vi "NATS Client Integration Test.vi"() -> (0 "error out":errorcluster)   [LabVIEW 2024]
uses:
  <vilib>/addons/_JKI Toolkits/Caraya/classes/Assert/Assert False.vi
  <vilib>/addons/_JKI Toolkits/Caraya/classes/Assert/Assert Equal Value and Type_Variant.vi
  NATS Subscription/NATS Subscription.lvclass
  <vilib>/addons/_JKI Toolkits/Caraya/classes/Test/Test.lvclass
  NATS Client/NATS Client.lvclass
  <vilib>/addons/_JKI Toolkits/Caraya/classes/Assert/Assert.lvclass
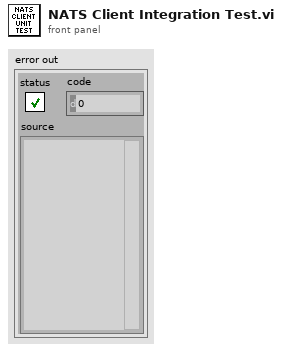
[diagram p1: front panel]
types:
  T1 = typedef "NATS Core.lvlib/nats message.ctl" = cluster{"subject":string, "payload":string, "sub id":string, "reply-to":string, "headers":string, "type":T2, "received":timestamp}
  T2 = typedef "NATS Core.lvlib/msg type.ctl" = enum16{"Undefined", "MSG", "HMSG", "+OK", "PING", "PONG", "-ERR", "INFO"}
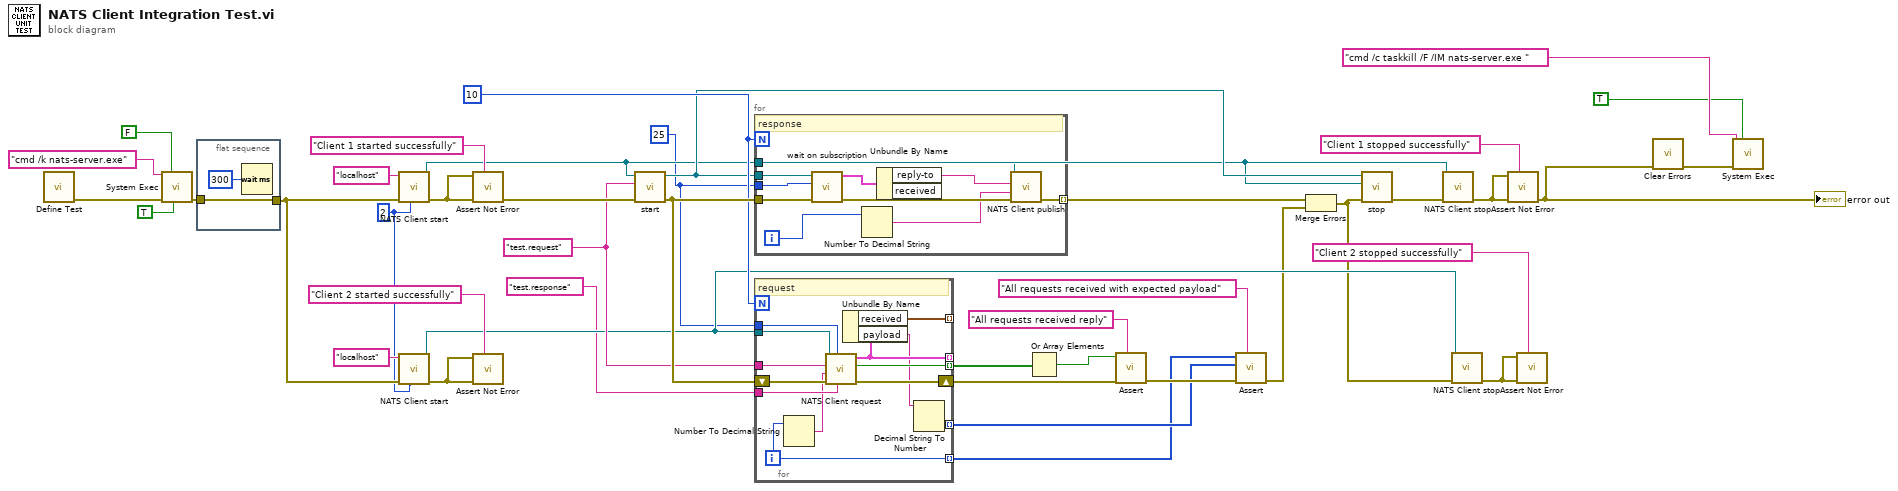
[diagram p0: block diagram]
diagram:
  w2 = 2 ("timeout ms (5)")
  w1 = 25 ("timeout in ms (-1)")
  w21 = 10
  w22 = "test.request"
  n1 = call <vilib>:"Define Test.vi"() -> ("error out"=w40:errorcluster)  [unwired: 10 in, 1 out]
  n2 = call <vilib>:"System Exec.vi"("run minimized? (F)"=TRUE, "wait until completion? (T)"=FALSE, "error in (no error)"=w40, "command line"="cmd /k nats-server.exe") -> ("error out"=w17:errorcluster)  [unwired: 4 in, 3 out]
  n3 = flat-sequence {
    tunnel: [w43] -> w16
    tunnel: w17 -> [w43]
    frame #0 {
      n4 = Wait (ms)(milliseconds to wait=u32 300) -> ()  [unwired: 1 out]
    }
  }
  n5 = call "NATS Client start.vi"("timeout ms (5)"=w2, "error in"=w16, "address"="localhost") -> ("error out"=w42:errorcluster, "NATS Client out"=w14:refnum<class "NATS Client.lvclass">)  [unwired: 7 in]
  n6 = call "NATS Client start.vi"("timeout ms (5)"=w2, "error in"=w16, "address"="localhost") -> ("error out"=w37:errorcluster, "NATS Client out"=w18:refnum<class "NATS Client.lvclass">)  [unwired: 7 in]
  n7 = call <vilib>:"Assert Not Error.vi"("Label"="Client 1 started successfully", "error in (no error)"=w42, "Not Error?"=w42) -> ("error out"=w36:errorcluster)  [unwired: 7 in, 1 out]
  n8 = call <vilib>:"Assert Not Error.vi"("Label"="Client 2 started successfully", "error in (no error)"=w37, "Not Error?"=w37) -> ()  [unwired: 7 in, 2 out]
  n9 = call "start.vi"("error in"=w36, "subject"=w22, "NATS Client"=w14) -> ("error out"=w33:errorcluster, "NATS Subscription"=w20:refnum<class "NATS Subscription.lvclass">)  [unwired: 7 in]
  n10 = for {
    N: w21 -> [_]
    tunnel: w20 -> [w53]
    tunnel: w14 -> [w51]
    tunnel: w1 -> [w45]
    tunnel: w33 -> [w54]
    tunnel: [w46] -> w11 mode=indexing
    i -> [w48]
    # "response"
    n11 = call-dynamic "wait on subscription.vi"("error in"=w54, "timeout in ms (-1)"=w45, "NATS Subscriber in"=w53) -> ("error out"=w52:errorcluster, "nats message"=w50:T1)  [unwired: 6 in, 1 out]
    n12 = Number To Decimal String(number=w48) -> (decimal integer string=w47:string)  [unwired: 1 in]
    n13 = Unbundle By Name(w50) -> ("reply-to"=w49:string)  [unwired: 1 out]
    n14 = call "NATS Client publish.vi"("error in"=w52, "payload"=w47, "subject"=w49, "NATS Client.lvlib:NATS Client.lvclass"=w51) -> ("error out"=w46:errorcluster)  [unwired: 7 in]
  }
  n15 = for {
    N: w21 -> [_]
    tunnel: w18 -> [w65]
    tunnel: w22 -> [w64]
    shift-right: [w66] -> w9
    shift-left: w33 -> [w67]
    tunnel: "test.response" -> [w63]
    tunnel: [w62] -> w13 mode=indexing
    tunnel: [w61] -> _ mode=indexing
    tunnel: [w58] -> w7 mode=indexing
    tunnel: [w57] -> w6 mode=indexing
    tunnel: [w56] -> _ mode=indexing
    tunnel: w1 -> [w55]
    i -> [w57]
    # "request"
    n16 = Number To Decimal String(number=w57) -> (decimal integer string=w60:string)  [unwired: 1 in]
    n17 = call "NATS Client request.vi"("reply subject"=w63, "timeout in ms (-1)"=w55, "error in"=w67, "payload"=w60, "subject"=w64, "NATS Client in"=w65) -> ("error out"=w66:errorcluster, "time out"=w62:bool, "nats message"=w61:T1)  [unwired: 3 in]
    n18 = Unbundle By Name(w61) -> ("received"=w56:timestamp, "payload"=w59:string)
    n19 = Decimal String To Number(string=w59) -> (number=w58:i32)  [unwired: 2 in, 1 out]
  }
  n20 = Or Array Elements(Boolean array=w13) -> (logical OR=w12:bool)
  n21 = call-poly <vilib>:"Assert.vi"("Label"="All requests received reply", "error in (no error)"=w9, "False?"=w12) -> ("error out"=w10:errorcluster)  [unwired: 7 in, 1 out]
  n22 = call-poly <vilib>:"Assert.vi"("Label"="All requests received with expected payload", "error in (no error)"=w10, "Y"=w7, "X"=w6) -> ("error out"=w4:errorcluster)  [unwired: 6 in, 1 out]
  n23 = Merge Errors(w11, w4) -> (w3:errorcluster)
  n24 = call "stop.vi"("error in"=w3, "NATS Client"=w14, "NATS Subscription"=w20) -> ("error out"=w35:errorcluster)  [unwired: 8 in]
  n25 = call "NATS Client stop.vi"("error in"=w35, "NATS Client"=w14) -> ("error out"=w41:errorcluster)  [unwired: 9 in]
  n26 = call "NATS Client stop.vi"("error in"=w3, "NATS Client"=w18) -> ("error out"=w34:errorcluster)  [unwired: 9 in]
  n27 = call <vilib>:"Assert Not Error.vi"("Label"="Client 1 stopped successfully", "error in (no error)"=w41, "Not Error?"=w41) -> ("error out"=w39:errorcluster)  [unwired: 7 in, 1 out]
  "error out" <- w39
  n28 = call <vilib>:"Assert Not Error.vi"("Label"="Client 2 stopped successfully", "error in (no error)"=w34, "Not Error?"=w34) -> ()  [unwired: 7 in, 2 out]
  n29 = call <vilib>:"Clear Errors.vi"("error in (no error)"=w39) -> ("error out"=w38:errorcluster)  [unwired: 5 in, 1 out]
  n30 = call <vilib>:"System Exec.vi"("wait until completion? (T)"=TRUE, "error in (no error)"=w38, "command line"="cmd /c taskkill /F /IM nats-server.exe ") -> ()  [unwired: 5 in, 4 out]
